vi "Boolean Decoder.vi"(1 "array":u8[](array[numeric]) format="%02x", 3 "Key":i32, 5 "error in (no error)":errorcluster) -> (15 "array w/ subset deleted":u8[](array[numeric]), 17 "Bool":bool, 19 "error out":errorcluster)   [LabVIEW 2023, in "Referee.lvclass"]
uses:
  Referee.lvclass
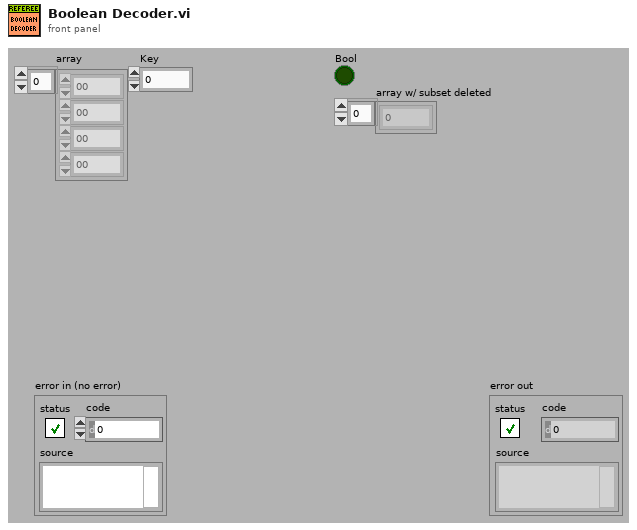
[diagram p1: front panel]
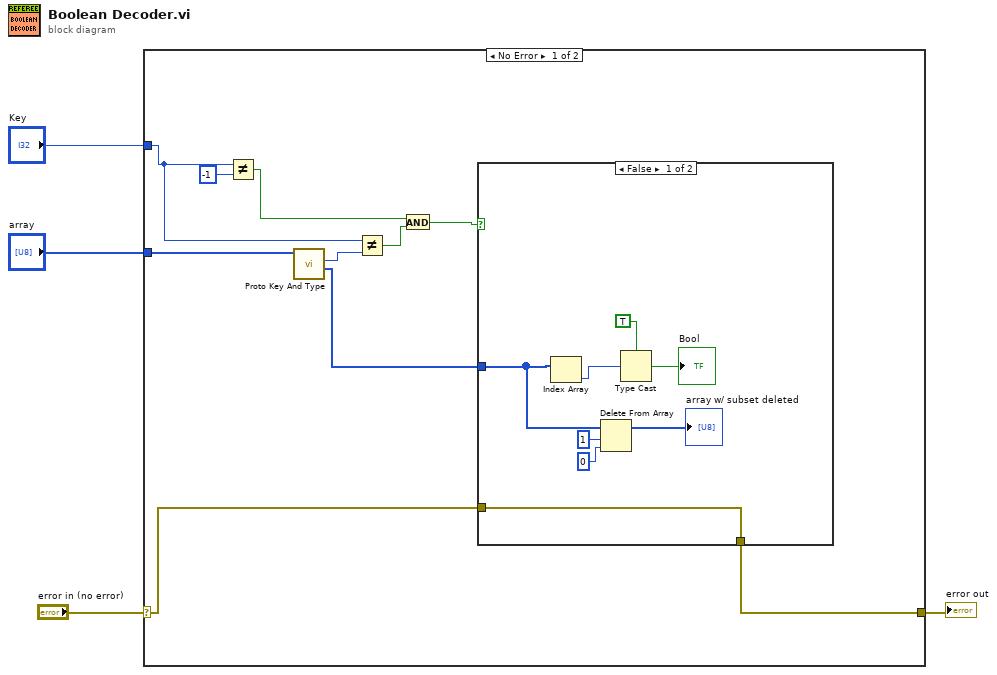
[diagram p0: block diagram]
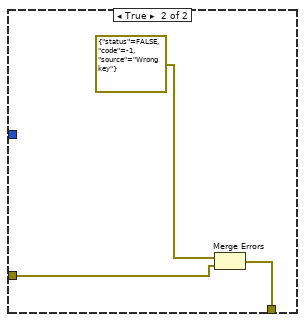
[diagram p2: hidden frame]
diagram:
  n1 = case shown="No Error" "error in (no error)" {
    selector: "error in (no error)" -> [w5 w26]
    tunnel: [w6 w26] -> w3
    tunnel: "array" -> [w14 _]
    tunnel: "Key" -> [w9 _]
    frame No Error {
      n2 = Not Equal?(x=w9, y=-1) -> (x != y?=w12:bool)
      n3 = call "Proto Key And Type.vi"("Array"=w14) -> ("array w/ subset deleted"=w7:u8[], "Key"=w10:i32)  [unwired: 8 in, 1 out]
      n4 = Not Equal?(x=w9, y=w10) -> (x != y?=w11:bool)
      n5 = And(x=w12, y=w11) -> (x .and. y?=w8:bool)
      n6 = case shown="False" w8 {
        tunnel: w7 -> [w16 _]
        tunnel: [w20 w23] -> w6
        tunnel: w5 -> [w20 w24]
        frame False {
          n7 = Index Array(array=w16) -> (element=w15:u8)  [unwired: 1 in]
          n8 = Delete From Array(array=w16, length=1, index=0) -> (array with subset deleted=→"array w/ subset deleted":u8[])  [unwired: 1 out]
          n9 = Type Cast(type=TRUE, x=w15) -> (*(type *) &x=→"Bool":bool)
        }
        frame True {
          n10 = Merge Errors(errorcluster {"status"=FALSE, "code"=-1, "source"="Wrong key"} ("error IO"), w24) -> (w23:errorcluster)
        }
      }
    }
    frame Error {
    }
  }
  "error out" <- w3
